vi "initialize Session Data.vi"(0 "OBJ - Session in":refnum<class "Text Device Session.lvclass">, 11 "error in":errorcluster) -> (4 "OBJ - Session out":refnum<class "Text Device Session.lvclass">, 15 "error out":errorcluster)   [LabVIEW 2019, in "Text Device Session.lvclass"]
doc: "OVERRIDE VI\nPlaceholder for decendant sessions to initialize and set their default values"
uses:
  Text Device Session.lvclass
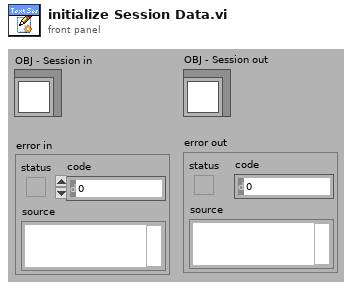
[diagram p1: front panel]
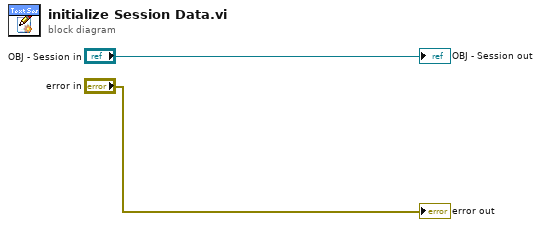
[diagram p0: block diagram]
diagram:
  "error out" <- "error in"
  "OBJ - Session out" <- "OBJ - Session in"
